vi "Write To Lights.vi"   [LabVIEW 2014]
uses:
  Common Code/Elevator State.ctl
  Common Code/Elevator Mode.ctl
  Robot Global Data.vi
types:
  T1 = typedef "Elevator Mode.ctl" = enum16{"Manual", "Safe", "Auto"}
  T2 = typedef "Elevator State.ctl" = enum16{"Idle", "Goto Load Position", "Wait for Load", "Load Drop", "Load Lift", "Drop Stack", "Goto Eject Position", "Eject ", "Raise Trashcan", "Open Stabilizer", "Untip Drop", "Untip Wait", "Untip Lift", "Abort Load", "HP Load Wait", "HP Load Drop", "HP Load Lift", "HP Load Abort", "Close Stabilizer", "HP Load Unfinish", "HP Load Score", "HP Load Finish", "HP Goto Finish Down", "HP Goto Finish Up", "Full"}
  T3 = typedef "Elevator Status.ctl" = cluster{"Height":dbl, "Enc Value":dbl, "Limit Override":bool, "Mode":T1, "High IR":bool, "Motor Out":dbl, "Ping Detect":bool, "Auto Elevator Indicators":T4, "Master Current":dbl, "Slave Current":dbl, "High Current":bool, "Current Tripped":bool, "Top Limit":bool, "Bottom Limit":bool, "Eject Piston":bool, "Stabilizer":bool, "Finger":bool, "Finger Height":dbl, "Finger Raw":dbl, "Finger at Bottom":bool}
  T4 = typedef "Auto Elevator Indicators.ctl" = cluster{"Target Out":dbl, "Storing Trashcan?":bool, "State":T2, "In Range":bool, "Store Can Command":bool, "HP Load":bool}
  T5 = typedef "WPI_DriverStationRobotMode2.ctl" = enum16{"Autonomous Disabled", "Autonomous Enabled", "Teleop Disabled", "Teleop Enabled", "Disconnected", "Finish", "Test Disabled", "Test Enabled", "Emergency Stopped"}
  T6 = typedef "Dashboard Control Data.ctl" = cluster{"Cam Exposure":dbl, "Go to angle":dbl, "Steer PID Gains":cluster{"proportional gain (Kc)":dbl, "integral time (Ti, min)":dbl, "derivative time (Td, min)":dbl}, "Steer PID output Range":cluster{"output high":dbl, "output low":dbl}, "Pressure m \nValue":dbl, "Pressure b \nValue":dbl, "Roller Command Cluster ":T7, "Elevator":T8, "Encoder Control":T10, "Auton Settings":cluster{"Drive Dist Window Size":dbl}, "Drivetrain Settings":T11, "Lance":T12}
  T7 = typedef "Roller Control.ctl" = cluster{"Intake Speed":dbl, "Turn In Speed":dbl, "Unload Speed":dbl, "Turn Out Speed":dbl, "Ping Align Tolerance":dbl, "Tote Range Threshold":dbl, "Right Pot 0":dbl, "Pot Threshold":dbl, "Left Pot 0":dbl, "Right Pot Scale":dbl, "Left Pot Scale":dbl, "Min Elevator Height":dbl, "Eject Time":dbl, "Eject US Threshold":dbl, "Anti-Twitch Time":u32, "Ping Caring Threshold":dbl, "Pot Diff Threshold":dbl, "Pinch Sustain":u32, "Absorb Give Up Threshold":dbl, "Untip In Threshold":dbl, "Untip Grab Range":dbl, "Ultrasonic Hold Time":u32, "Landscape Absorb Time":u32, "Pot Use Wait Time":u32, "Can Turn Stop Range":dbl, "HP Load Speed":dbl, "Stick Multiplier":dbl}
  T8 = typedef "Elevator DB Control.ctl" = cluster{"PID Output Range":cluster{"output high":dbl, "output low":dbl}, "PID gains":cluster{"proportional gain (Kc)":dbl, "integral time (Ti, min)":dbl, "derivative time (Td, min)":dbl}, "Height Tolerance":sgl, " Encoder Constant":dbl, "Eject Time":sgl, "Zeroing Speed":sgl, "Presets":T9, "Ping Detect Threshold":sgl, "Trashcan Detect Threshold":sgl, "Zero Filter Time":dbl, "Stabilizer Open Time":dbl, "Zero Creep Speed":dbl, "Max Current":dbl, "Current Trip Time":dbl, "Abort Pitch":dbl, "Finger m":dbl, "Finger b":dbl, "Finger max ":dbl, "Finger Stabilizer":dbl, "Finger Store":dbl, "Finger Stop Store":dbl, "Stabilizer Close Time":dbl, "Finger min":dbl, "Unstick gain":dbl}
  T9 = typedef "Elevator Presets.ctl" = cluster{"Pickup 2 w/ Tote":sgl, "Pickup 2 w/ Trashcan":sgl, "Pickup 3 w/ Tote":sgl, "Pickup 3 w/ Trashcan":sgl, "Bottom":sgl, "Pickup 1 w/ Tote":sgl, "Pickup Trashcan":sgl, "Pickup 1 w/ Trashcan":sgl, "Eject":sgl, "Hold Low":sgl, "Step add height":sgl, "Untip Lift":dbl, "Drop Stack":dbl, "HP Load Hold":dbl, "HP Load Drop":dbl, "HP Load Hold Can":dbl, "Store can max":dbl, "HP Drag Score":dbl, "HP Drag Finish":dbl, "Finger trashcan avoid":dbl, "Full":dbl}
  T10 = typedef "Encoder Control.ctl" = cluster{"Left Tick Constant":dbl, "Right Tick Constant":dbl, "Center Tick Constant":dbl, "Reset?":bool, "Y Dist":cluster{"PID gains":cluster{"proportional gain (Kc)":dbl, "integral time (Ti, min)":dbl, "derivative time (Td, min)":dbl}}, "X Dist":cluster{"PID gains":cluster{"proportional gain (Kc)":dbl, "integral time (Ti, min)":dbl, "derivative time (Td, min)":dbl}}, "Y Stop Thresh":dbl, "Y Stop Speed":dbl, "X Stop Thresh":dbl, "X Stop Speed":dbl}
  T11 = typedef "Drivetrain Settings.ctl" = cluster{"Gyro Tolerance":sgl, "Strafe Correct max steer":sgl, "Strafe Timer Wait":sgl, "Throttle Ramp (ms)":sgl, "Strafe Ramp (ms)":sgl, "Angular rate compensation":bool, "Throttle to Rate Scale":sgl, "Rate compensation gain":sgl, "Creep Steer":sgl, "Creep Throttle":sgl}
  T12 = typedef "Pike DB Controls.ctl" = cluster{"Down Speed":dbl, "Up Speed":dbl, "Max Down Time":dbl, "Max Up Time":dbl, "Current Limit":dbl}
  T13 = typedef "WPI_DriverStationAllianceInfo.ctl" = enum16{"Red", "Blue", "Invalid"}
  T14 = typedef "WPI_DigitalOutputDevRef.ctl" = cluster{"Controller":T15, "DIO Channel":T16, "DevStatus":errorcluster}
  T15 = typedef "FPGA_TypedefDigitalModule.ctl" = enum16{"Controller 1"}
  T16 = typedef "FPGA_DIOChannel.ctl" = enum8{"DIO 0", "DIO 1", "DIO 2", "DIO 3", "DIO 4", "DIO 5", "DIO 6", "DIO 7", "DIO 8", "DIO 9", "DIO MXP 0", "DIO MXP 1", "DIO MXP 2", "DIO MXP 3", "DIO MXP 4", "DIO MXP 5", "DIO MXP 6", "DIO MXP 7", "DIO MXP 8", "DIO MXP 9", "DIO MXP 10", "DIO MXP 11", "DIO MXP 12", "DIO MXP 13", "DIO MXP 14", "DIO MXP 15", "Invalid"}
  T17 = typedef "WPI_AOChannelDevRef.ctl" = cluster{"DevStatus":errorcluster, "Controller":T18, "AO Channel":T19}
  T18 = typedef "FPGA_TypedefAnalogModule.ctl" = enum16{"Controller 1"}
  T19 = typedef "WPI_AnalogOutputChannel.ctl" = enum8{"AO MXP 0", "AO MXP 1", "Invalid"}
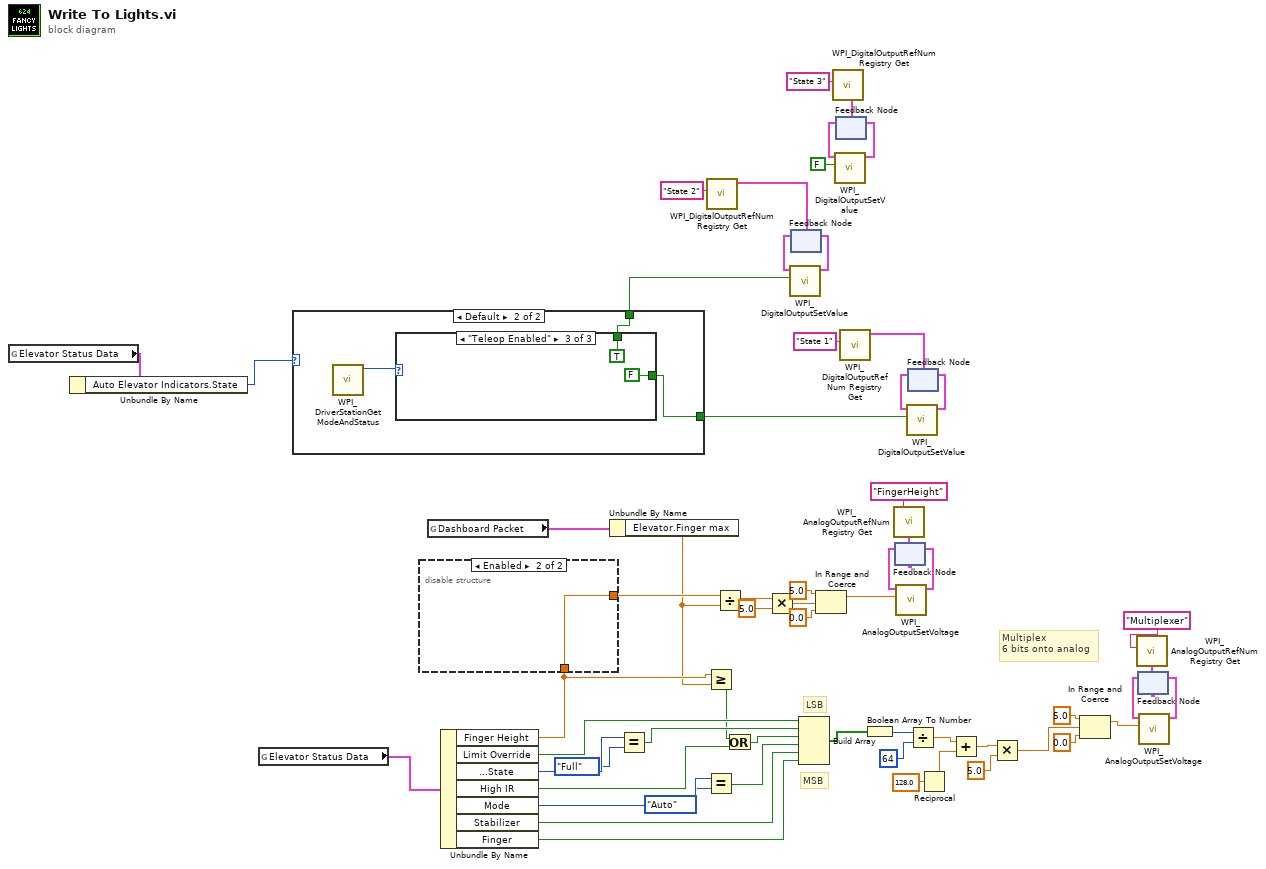
[diagram p0: block diagram]
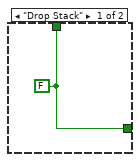
[diagram p2: hidden frame]
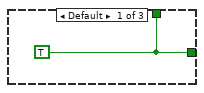
[diagram p3: hidden frame]
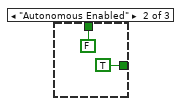
[diagram p4: hidden frame]
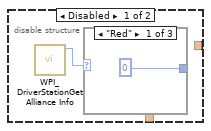
[diagram p5: hidden frame]
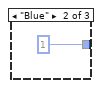
[diagram p6: hidden frame]
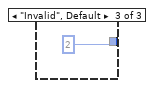
[diagram p7: hidden frame]
diagram:
  # "MSB"
  # "LSB"
  # "Multiplex\n6 bits onto analog"
  n1 = global read "Robot Global Data.vi" "Elevator Status Data"() -> (w32:T3)
  n2 = Unbundle By Name(w32) -> ("Auto Elevator Indicators.State"=w31:T2)
  n3 = global read "Robot Global Data.vi" "Elevator Status Data"() -> (w60:T3)
  n4 = case shown="Default" w31 {
    tunnel: [w61 w63] -> w30
    tunnel: [w61 w62] -> w29
    frame "Drop Stack" {
      w61 = FALSE
    }
    frame Default {
      n5 = call <vilib>:"WPI_DriverStationGetModeAndStatus.vi"() -> ("Robot Mode"=w64:T5)  [unwired: 10 in, 1 out]
      n6 = case shown="\"Teleop Enabled\"" w64 {
        tunnel: [w65 TRUE FALSE] -> w63
        tunnel: [w65 FALSE TRUE] -> w62
        frame Default {
          w65 = TRUE
        }
        frame "Autonomous Enabled" {
        }
        frame "Teleop Enabled" {
        }
      }
    }
  }
  n7 = global read "Robot Global Data.vi" "Dashboard Packet"() -> (w51:T6)
  n8 = Unbundle By Name(w60) -> ("Finger Height"=w22:dbl, "Limit Override"=w26:bool, "Auto Elevator Indicators.State"=w25:T2, "High IR"=w19:bool, "Mode"=w28:T1, "Stabilizer"=w15:bool, "Finger"=w14:bool)
  n9 = disable-structure shown="Enabled" {
    disable-tunnel: w22 -> [_ w74]
    disable-tunnel: [_ w74] -> w50
    frame Disabled {
      n10 = call <vilib>:"WPI_DriverStationGet Alliance Info.vi"() -> ("Alliance"=w70:T13)  [unwired: 10 in, 1 out]
      n11 = case shown="\"Red\"" w70 {
        tunnel: [u8 0 u8 1 u8 2 ("I2CRegister")] -> _
        frame "Red" {
        }
        frame "Blue" {
        }
        frame "Invalid", Default {
        }
      }
    }
    frame Enabled {
    }
  }
  n12 = Unbundle By Name(w51) -> ("Elevator.Finger max"=w21:dbl)
  n13 = Equal?(x=w25, y=Elevator_State."Full") -> (x = y?=w23:bool)
  n14 = Greater Or Equal?(x=w22, y=w21) -> (x >= y?=w20:bool)
  n15 = Equal?(x=w28, y=Elevator_Mode."Auto") -> (x = y?=w16:bool)
  n16 = call <vilib>:"WPI_DigitalOutputRefNum Registry Get.vi"("refnum name"="State 2") -> ("DigitalOutputDevRef"=w33:T14)  [unwired: 9 in, 1 out]
  n17 = Divide(x=w50, y=w21) -> (x/y=w49:dbl)
  n18 = Or(x=w20, y=w19) -> (x .or. y?=w18:bool)
  n19 = Multiply(x=w49, y=5.0) -> (x*y=w47:dbl)
  n20 = feedback #1(w33) -> (w35:T14)
  n21 = call <vilib>:"WPI_DigitalOutputSetValue.vi"("Value"=w29, "DigitalOutputDevRef"=w35) -> ("DigitalOutputDevRef"=w34:T14)  [unwired: 8 in, 1 out]
  n22 = feedback-in #1(w34) -> ()
  n23 = Build Array(w26, w23, w18, w16, w15, w14) -> (w27:bool[])
  n24 = In Range and Coerce(upper limit=5.0, x=w47, lower limit=0.0) -> (coerced(x)=w44:dbl)  [unwired: 1 out]
  n25 = call <vilib>:"WPI_DigitalOutputRefNum Registry Get.vi"("refnum name"="State 3") -> ("DigitalOutputDevRef"=w5:T14)  [unwired: 9 in, 1 out]
  n26 = feedback #2(w5) -> (w4:T14)
  n27 = call <vilib>:"WPI_DigitalOutputSetValue.vi"("Value"=FALSE, "DigitalOutputDevRef"=w4) -> ("DigitalOutputDevRef"=w1:T14)  [unwired: 8 in, 1 out]
  n28 = feedback-in #2(w1) -> ()
  n29 = call <vilib>:"WPI_DigitalOutputRefNum Registry Get.vi"("refnum name"="State 1") -> ("DigitalOutputDevRef"=w58:T14)  [unwired: 9 in, 1 out]
  n30 = Boolean Array To Number(Boolean array=w27) -> (number=w13:u32)
  n31 = call <vilib>:"WPI_AnalogOutputRefNum Registry Get.vi"("refnum name"="FingerHeight") -> ("AODeviceRef"=w54:T17)  [unwired: 9 in, 1 out]
  n32 = feedback #3(w54) -> (w53:T17)
  n33 = call <vilib>:"WPI_AnalogOutputSetVoltage.vi"("Voltage"=w44, "AODeviceRef"=w53) -> ("AODeviceRef"=w52:T17)  [unwired: 8 in, 1 out]
  n34 = feedback-in #3(w52) -> ()
  n35 = feedback #4(w58) -> (w56:T14)
  n36 = call <vilib>:"WPI_DigitalOutputSetValue.vi"("Value"=w30, "DigitalOutputDevRef"=w56) -> ("DigitalOutputDevRef"=w57:T14)  [unwired: 8 in, 1 out]
  n37 = feedback-in #4(w57) -> ()
  n38 = Divide(x=w13, y=u32 64) -> (x/y=w11:dbl)
  n39 = Reciprocal(x=128.0) -> (1/x=w10:dbl)
  n40 = Add(x=w11, y=w10) -> (x+y=w8:dbl)
  n41 = Multiply(x=w8, y=5.0) -> (x*y=w6:dbl)
  n42 = In Range and Coerce(upper limit=5.0, x=w6, lower limit=0.0) -> (coerced(x)=w39:dbl)  [unwired: 1 out]
  n43 = call <vilib>:"WPI_AnalogOutputRefNum Registry Get.vi"("refnum name"="Multiplexer") -> ("AODeviceRef"=w42:T17)  [unwired: 9 in, 1 out]
  n44 = feedback #5(w42) -> (w38:T17)
  n45 = call <vilib>:"WPI_AnalogOutputSetVoltage.vi"("Voltage"=w39, "AODeviceRef"=w38) -> ("AODeviceRef"=w43:T17)  [unwired: 8 in, 1 out]
  n46 = feedback-in #5(w43) -> ()
